vi "Global-Stop (SubVI).vi"(1 "Mode (Read)":enum16{"Read", "Write"}(ring), 3 "IN":bool) -> (0 "OUT":bool)   [LabVIEW 2012]
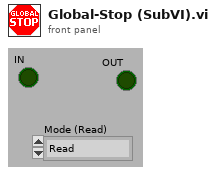
[diagram p1: front panel]
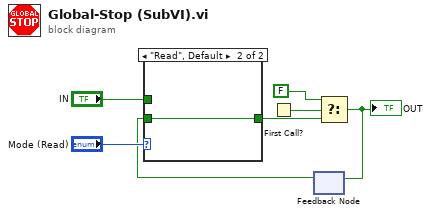
[diagram p0: block diagram]
diagram:
  n1 = First Call?() -> (First Call?: T/F=w3:bool)
  n2 = feedback #1() -> (w5:bool)  [unwired: 1 in]
  n3 = case shown="\"Read\", Default" "Mode (Read)" {
    tunnel: [w8 w9] -> w2
    tunnel: w5 -> [_ w9]
    tunnel: "IN" -> [w8 _]
    frame "Write" {
    }
    frame "Read", Default {
    }
  }
  n4 = Select(t=FALSE ("IN"), s=w3, f=w2) -> (s? t:f=w1:bool)
  "OUT" <- w1
  n5 = feedback-in #1(w1) -> ()
